vi "PQ Example Many INSERTs.vi"() -> ()   [LabVIEW 2016]
uses:
  Result/PQ Result.lvclass/PQ Result.ctl
  Connection/Execute Command (No results).vi
  Result/Clear.vi
  Connection/Execute Command (Result).vi
  Connection/Execute (no results).vi
  Connection/Execute (Return first result with rows).vi
  Connection/Single Command with parameters.vi
  Connection/PQ Connection.lvclass
panel:
  in  "Connection Strings to access PostgreSQL":string="host=localhost port=5432 dbname = mydb "
  out "INSERTS/sec":dbl format="%#_3p"
  out "Time per INSERT":dbl format="%#_3p"
  out "error out":errorcluster
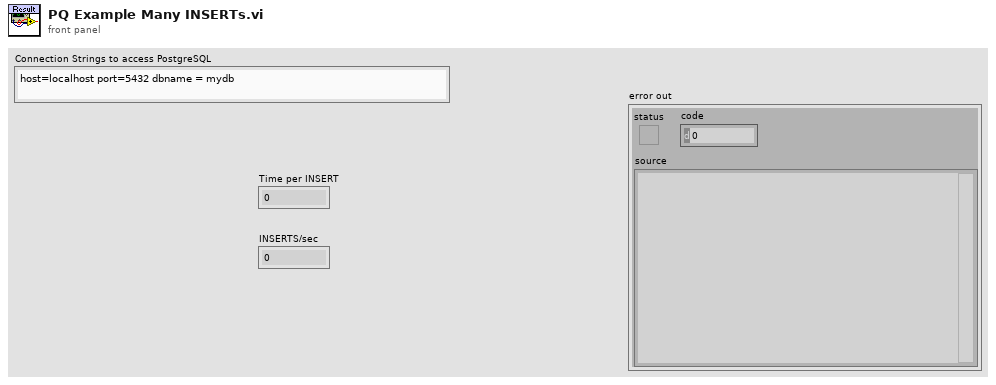
[diagram p1: front panel]
types:
  T1 = cluster{cluster{i32, "number: 0 to 1":dbl, string}, "seconds since 1Jan1904":timestamp}
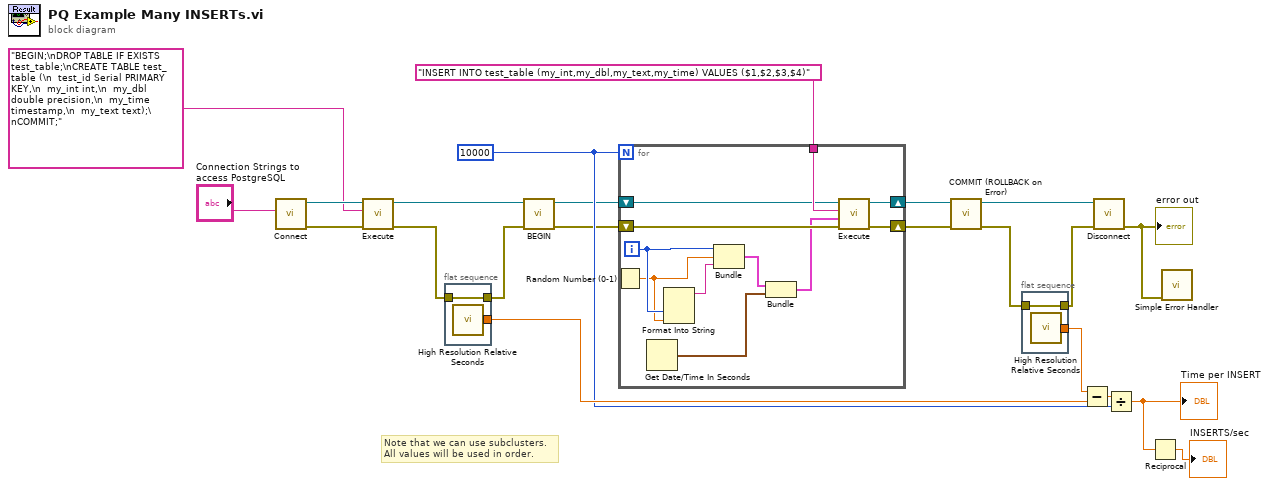
[diagram p0: block diagram]
diagram:
  w6 = 10000
  # "Note that we can use subclusters.\nAll values will be used in order."
  n1 = call "Connect.vi"("Connection Strings"="Connection Strings to access PostgreSQL") -> ("error out"=w16:errorcluster, "PQ Connection out"=w18:refnum<class "PQ Connection.lvclass">)  [unwired: 9 in]
  n2 = call-poly "Execute.vi"("error in (no error)"=w16, "SQL"="BEGIN;\nDROP TABLE IF EXISTS test_table;\nCREATE TABLE test_table (\n  test_id Serial PRIMARY KEY,\n  my_int int,\n  my_dbl double precision,\n  my_time timestamp,\n  my_text text);\nCOMMIT;", "PQ Connection in"=w18) -> ("error out"=w12:errorcluster, "PQ Connection out"=w17:refnum<class "PQ Connection.lvclass">)  [unwired: 7 in]
  n3 = flat-sequence {
    tunnel: w12 -> [w24]
    tunnel: [w24] -> w4
    tunnel: [w23] -> w8
    frame #0 {
      n4 = call <vilib>:"High Resolution Relative Seconds.vi"() -> ("relative seconds"=w23:dbl)
    }
  }
  n5 = call "BEGIN.vi"("error in (no error)"=w4, "PQ Connection in"=w17) -> ("error out"=w3:errorcluster, "PQ Connection out"=w5:refnum<class "PQ Connection.lvclass">)  [unwired: 8 in]
  n6 = for {
    N: w6 -> [_]
    tunnel: "INSERT INTO test_table (my_int,my_dbl,my_text,my_time) VALUES ($1,$2,$3,$4)" ("command") -> [w34]
    shift-right: [w35] -> w21
    shift-left: w5 -> [w33]
    shift-right: [w31] -> w13
    shift-left: w3 -> [w32]
    i -> [w30]
    n7 = Random Number (0-1)() -> (number: 0 to 1=w29:dbl)
    n8 = Get Date/Time In Seconds() -> (seconds since 1Jan1904=w25:timestamp)
    n9 = Format Into String(w30, w29) -> (resulting string=w28:string)  [unwired: 3 in, 1 out]
    n10 = Bundle(w30, "number: 0 to 1"=w29, w28) -> (w26:cluster{i32, "number: 0 to 1":dbl, string})  [unwired: 1 in]
    n11 = Bundle(w26, "seconds since 1Jan1904"=w25) -> (w27:T1)  [unwired: 1 in]
    n12 = call-poly "Execute.vi"("error in (no error)"=w32, "Parameters"=w27, "SQL"=w34, "PQ Connection in"=w33) -> ("error out"=w31:errorcluster, "PQ Connection out"=w35:refnum<class "PQ Connection.lvclass">)  [unwired: 6 in]
  }
  n13 = call "COMMIT (ROLLBACK on Error).vi"("error in (no error)"=w13, "PQ Connection in"=w21) -> ("error out"=w11:errorcluster, "PQ Connection out"=w14:refnum<class "PQ Connection.lvclass">)  [unwired: 8 in]
  n14 = flat-sequence {
    tunnel: w11 -> [w37]
    tunnel: [w37] -> w10
    tunnel: [w36] -> w9
    frame #0 {
      n15 = call <vilib>:"High Resolution Relative Seconds.vi"() -> ("relative seconds"=w36:dbl)
    }
  }
  n16 = Subtract(x=w9, y=w8) -> (x-y=w7:dbl)
  n17 = call-dynamic "Disconnect.vi"("error in (no error)"=w10, "PQ Connection in"=w14) -> ("error out"=w19:errorcluster)  [unwired: 9 in]
  "error out" <- w19
  n18 = Divide(x=w7, y=w6) -> (x/y=w2:dbl)
  "Time per INSERT" <- w2
  n19 = Reciprocal(x=w2) -> (1/x=→"INSERTS/sec":dbl)
  n20 = call <vilib>:"Simple Error Handler.vi"("error in (no error)"=w19) -> ()  [unwired: 4 in, 5 out]
